vi "XY Localizer Kalman Matrices.vi"(8 "dt (s)":dbl, 10 "State Estimate Standard Deviation":dbl, 11 "Sensors":T3[](array[typedef])) -> (3 "Dynamical System Matrices":T1)   [LabVIEW 2020]
uses:
  ctl/XY (Position-Velocity) Sensor Instance.ctl
  ctl/Dynamical System Matrices.ctl
  <vilib>/Analysis/Matrix/Datatypes/RealMatrix.ctl
  ctl/Dynamical System Templates.ctl
  <vilib>/Analysis/7linalg.llb/Create Special Real Matrix.vi
  <vilib>/Analysis/NI_AALPro.lvlib
  <vilib>/Analysis/Matrix/NI_Matrix.lvlib
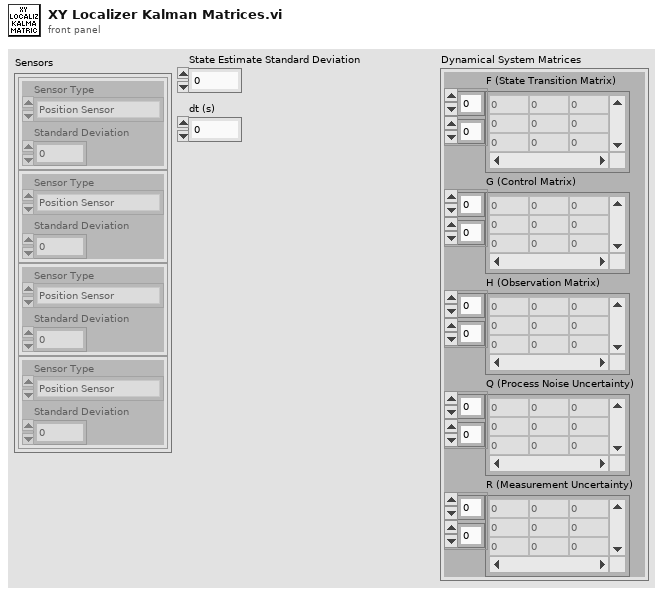
[diagram p1: front panel]
types:
  T1 = typedef "Dynamical System Matrices.ctl" = cluster{"F (State Transition Matrix)":T2, "G (Control Matrix)":T2, "H (Observation Matrix)":T2, "Q (Process Noise Uncertainty)":T2, "R (Measurement Uncertainty)":T2}
  T2 = typedef "NI_Matrix.lvlib/RealMatrix.ctl" = dbl[][]
  T3 = typedef "XY (Position-Velocity) Sensor Instance.ctl" = cluster{"Sensor Type":enum16{"Position Sensor", "Velocity Sensor"}, "Standard Deviation":dbl}
  T4 = typedef "Dynamical System Templates.ctl" = enum16{"XY Point Mass"}
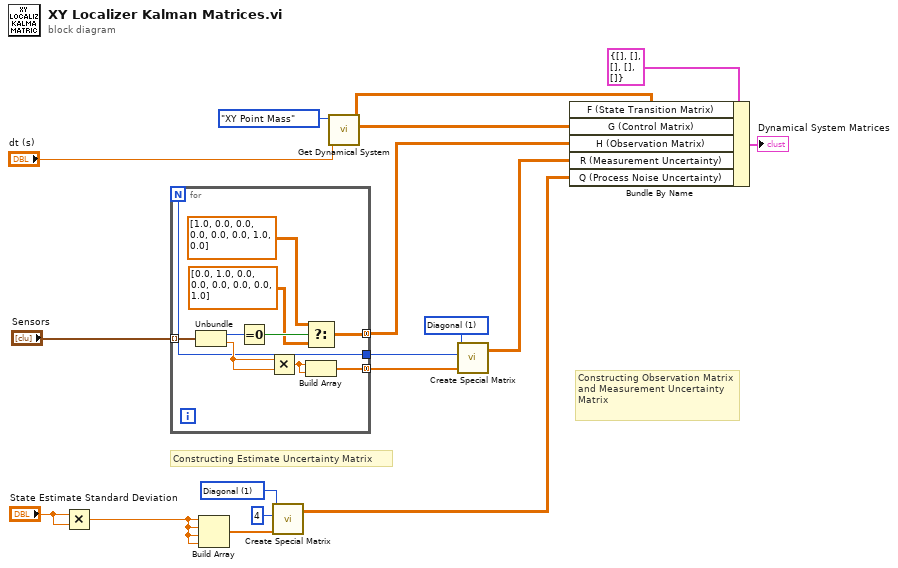
[diagram p0: block diagram]
diagram:
  w9 = 1 items=["Identity", "Diagonal", "Toeplitz", "Vandermonde", "Companion", "Hankel", "Hadamard", "Wilkinson", "Hilbert", "Inverse Hilbert", "Rosser", "Pascal"] ("matrix type")
  w5 = 1 items=["Identity", "Diagonal", "Toeplitz", "Vandermonde", "Companion", "Hankel", "Hadamard", "Wilkinson", "Hilbert", "Inverse Hilbert", "Rosser", "Pascal"] ("matrix type")
  # "Constructing Observation Matrix and Measurement Uncertainty Matrix"
  # "Constructing Estimate Uncertainty Matrix"
  n1 = Multiply(x="State Estimate Standard Deviation", y="State Estimate Standard Deviation") -> (x*y=w1:dbl)
  n2 = for {
    N -> [w19]
    tunnel: "Sensors" -> [w28] mode=indexing
    tunnel: [w23] -> w15 mode=concatenating
    tunnel: [w20] -> w10 mode=concatenating
    tunnel: [w19] -> w11
    n3 = Unbundle(w28) -> ("Sensor Type"=w27:enum16{"Position Sensor", "Velocity Sensor"}, "Standard Deviation"=w22:dbl)
    n4 = Equal To 0?(x=w27) -> (x = 0?=w26:bool)
    n5 = Multiply(x=w22, y=w22) -> (x*y=w21:dbl)
    n6 = Select(t=T2 [[1.0, 0.0, 0.0, 0.0], [0.0, 0.0, 1.0, 0.0]] ("Special Matrix"), s=w26, f=T2 [[0.0, 1.0, 0.0, 0.0], [0.0, 0.0, 0.0, 1.0]] ("Special Matrix")) -> (s? t:f=w23:T2)
    n7 = Build Array(w21, w21) -> (w20:dbl[])
  }
  n8 = Build Array(w1, w1, w1, w1) -> (w6:dbl[])
  n9 = call-poly <vilib>:"Create Special Matrix.vi"("matrix type"=w5, "matrix size"=4, "Input Vector1"=w6) -> ("Special Matrix"=w16:T2)  [unwired: 2 in, 1 out]
  n10 = call "Get Dynamical System.vi"("dt"="dt (s)", "Dynamical System"=Dynamical_System_Templates."XY Point Mass") -> ("G (Control Input Matrix)"=w14:T2, "F (State Transition Matrix)"=w13:T2)  [unwired: 8 in]
  n11 = call-poly <vilib>:"Create Special Matrix.vi"("matrix type"=w9, "matrix size"=w11, "Input Vector1"=w10) -> ("Special Matrix"=w17:T2)  [unwired: 2 in, 1 out]
  n12 = Bundle By Name(cluster=T1 {"F (State Transition Matrix)"=[], "G (Control Matrix)"=[], "H (Observation Matrix)"=[], "Q (Process Noise Uncertainty)"=[], "R (Measurement Uncertainty)"=[]} ("Dynamical System Matrices"), "F (State Transition Matrix)"=w13, "G (Control Matrix)"=w14, "H (Observation Matrix)"=w15, "R (Measurement Uncertainty)"=w17, "Q (Process Noise Uncertainty)"=w16) -> (→"Dynamical System Matrices":T1)
